vi "DSF.Engine.Pool.Create.vi"(8 "error in (no error)":errorcluster, 10 "number of elements":u32, 11 "Pool type":refnum<class "DSF.Engine.Pool.lvclass">) -> (0 "error out":errorcluster, 3 "Pool":refnum<class "DSF.Engine.Pool.lvclass">)   [LabVIEW 2016, in "DSF.Engine.lvlib" / "DSF.Engine.Pool.lvclass"]
uses:
  DSF.Engine.Pool.lvclass
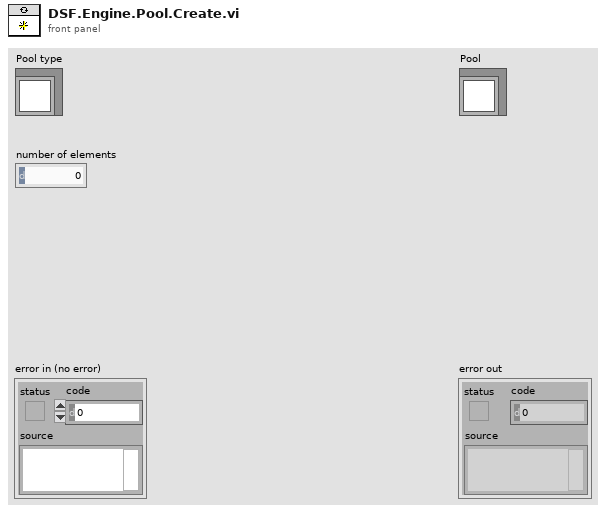
[diagram p1: front panel]
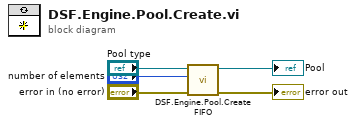
[diagram p0: block diagram]
diagram:
  n1 = call "DSF.Engine.Pool.Create FIFO.vi"("error in (no error)"="error in (no error)", "number of elements"="number of elements", "Pool in"="Pool type") -> ("error out"=→"error out":errorcluster, "Pool out"=→"Pool":refnum<class "DSF.Engine.Pool.lvclass">)  [unwired: 7 in]
